vi "Read Multiple Samples.vi"(0 "TDMS In":refnum<k34>, 7 "#samples (-1: all)":i64=-1, 11 "Error In":errorcluster) -> (4 "TDMS Out":refnum<k34>, 6 "Input Vectors":dbl[][](array[numeric]), 8 "Output Vectors":dbl[][](array[numeric]), 14 "EOF?":bool, 15 "Error Out":errorcluster)   [LabVIEW 2015, in "Teaching File.lvlib"]
doc: "Read multiple teaching samples from TDMS file. Input_Data and Output_Data are the groups read for the data.\n\nColumns represent the index of input or output and the rows represent each teaching sample. Both 2D arrays should have the same # of rows.\n\nChannel names are NOT used for ordering the columns. If you want to change ordering of columns modify the NI_ArrayColumn property for the groups. You can rename the channels to any descriptive name you need.\n\nIf end of file is reached, the Read_Index is set to 0, preparing for another read from the start of the file.\nIf the Input_Data or Output_Data don't exist, return EOF? = True"
uses:
  Teaching File.lvlib
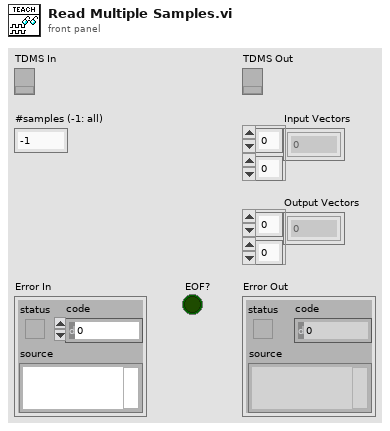
[diagram p1: front panel]
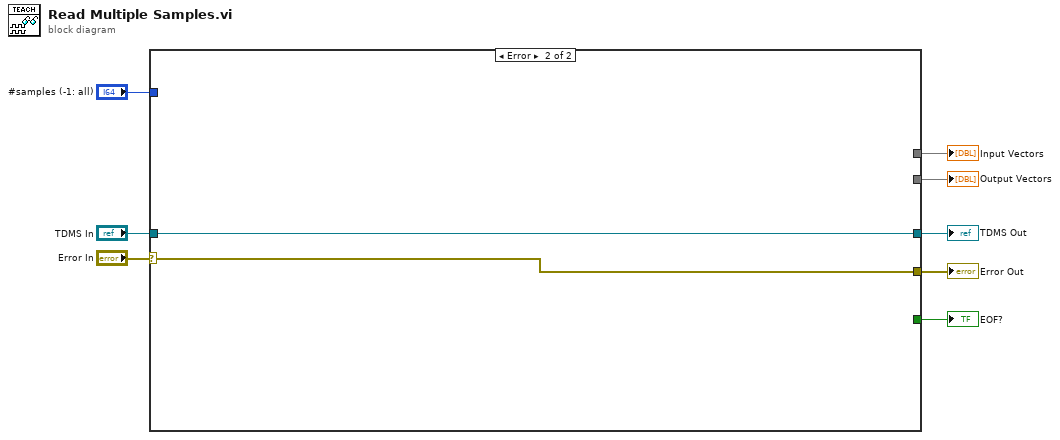
[diagram p0: block diagram]
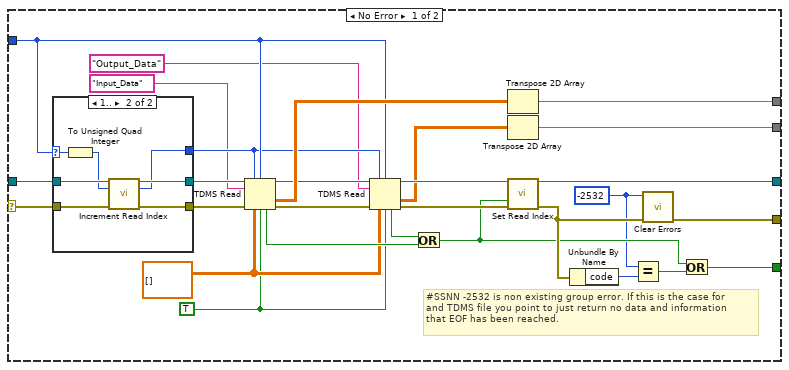
[diagram p2: hidden frame]
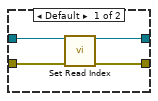
[diagram p3: hidden frame]
diagram:
  n1 = case shown="Error" "Error In" {
    selector: "Error In" -> [w11 w49]
    tunnel: "TDMS In" -> [w34 w48]
    tunnel: [w33 w48] -> w7
    tunnel: "#samples (-1: all)" -> [w29 _]
    tunnel: [w20 _] -> w5
    tunnel: [w19 _] -> w4
    tunnel: [w16 _] -> w3
    tunnel: [w12 w49] -> w2
    frame No Error {
      w13 = -2532 ("specific error code to clear (0: all)")
      w25 = TRUE ("return channels in file order? (F)")
      w26 = dbl[][] [] ("VectorData")
      # "#SSNN -2532 is non existing group error. If this is the case for \nand TDMS file you point to just return no data and information\nthat EOF has been reached."
      n2 = case shown="1.." w29 {
        selector: w29 -> [_ w42]
        tunnel: w11 -> [w39 w47]
        tunnel: [w37 w46] -> w36
        tunnel: [w38 w45] -> w35
        tunnel: [_ w44] -> w28
        tunnel: w34 -> [w40 w43]
        frame Default {
          n3 = call "Set Read Index.vi"("TDMS In"=w40, "Error In"=w39) -> ("TDMS Out"=w38:refnum<k34>, "Error Out"=w37:errorcluster)  [unwired: 12 in]
        }
        frame 1.. {
          n4 = To Unsigned Quad Integer(1:w42) -> (0:w41:u64)
          n5 = call "Increment Read Index.vi"("TDMS In"=w43, "Increment(1)"=w41, "Error In"=w47) -> ("TDMS Out"=w45:refnum<k34>, "Read Index"=w44:i64, "Error Out"=w46:errorcluster)  [unwired: 10 in]
        }
      }
      n6 = TDMS Read(0:w35, 1:w28, 2:w29, 5:"Input_Data" ("group name in"), 11:w36, 12:w26, 13:w25) -> (4:w31:refnum<k34>, 10:w32:dbl[][], 14:w27:bool, 15:w30:errorcluster)  [unwired: 1 in, 2 out]
      n7 = TDMS Read(0:w31, 1:w28, 2:w29, 5:"Output_Data" ("group name in"), 11:w30, 12:w26, 13:w25) -> (4:w23:refnum<k34>, 10:w21:dbl[][], 14:w24:bool, 15:w22:errorcluster)  [unwired: 1 in, 2 out]
      n8 = Or(x=w24, y=w27) -> (x .or. y?=w14:bool)
      n9 = Transpose 2D Array(2D array=w32) -> (transposed array=w19:dbl[][])
      n10 = Transpose 2D Array(2D array=w21) -> (transposed array=w20:dbl[][])
      n11 = call "Set Read Index.vi"("TDMS In"=w23, "Enable(True)"=w14, "Error In"=w22) -> ("TDMS Out"=w33:refnum<k34>, "Error Out"=w15:errorcluster)  [unwired: 11 in]
      n12 = Unbundle By Name(w15) -> ("code"=w18:i32)
      n13 = Equal?(x=w13, y=w18) -> (x = y?=w17:bool)
      n14 = call <vilib>:"Clear Errors.vi"("error in (no error)"=w15, "specific error code to clear (0: all)"=w13) -> ("error out"=w12:errorcluster)  [unwired: 4 in, 1 out]
      n15 = Or(x=w14, y=w17) -> (x .or. y?=w16:bool)
    }
    frame Error {
    }
  }
  "Error Out" <- w2
  "TDMS Out" <- w7
  "EOF?" <- w3
  "Input Vectors" <- w4
  "Output Vectors" <- w5
